vi "myRIO Main.vi"() -> ()   [LabVIEW 2014]
uses:
  Type Defs/VL6180X DEFS.ctl
  <vilib>/Analysis/baseanly.llb/Mean (DBL).vi
  <vilib>/MakerHub/LINX/Public/Utilities/Open Local.vi
  <vilib>/MakerHub/LINX/LMH-LINX.lvlib
  <vilib>/Analysis/NI_AALBase.lvlib
panel:
  in  "Speed Read":bool=TRUE
  out "Loop Rate (Hz)":u32
  in  "Offset":u8 format="%02x"
  out "Data out":u8 format="%02x"
  out "range":dbl
  out "Array":dbl[](array[numeric])
  out "min value":dbl
  out "max value":dbl
  in  "Samples to Avg":i32=10
  in  "milliseconds to wait":u32=20
  out "Sensor Error Code":u8
  in  "Stop":bool
  out "Distance":cluster{"Distance (mm)":u8, u8}(graph)
  # "0 = No error\n6 = early convergence estimate check failed\n7 = max convergence issue"
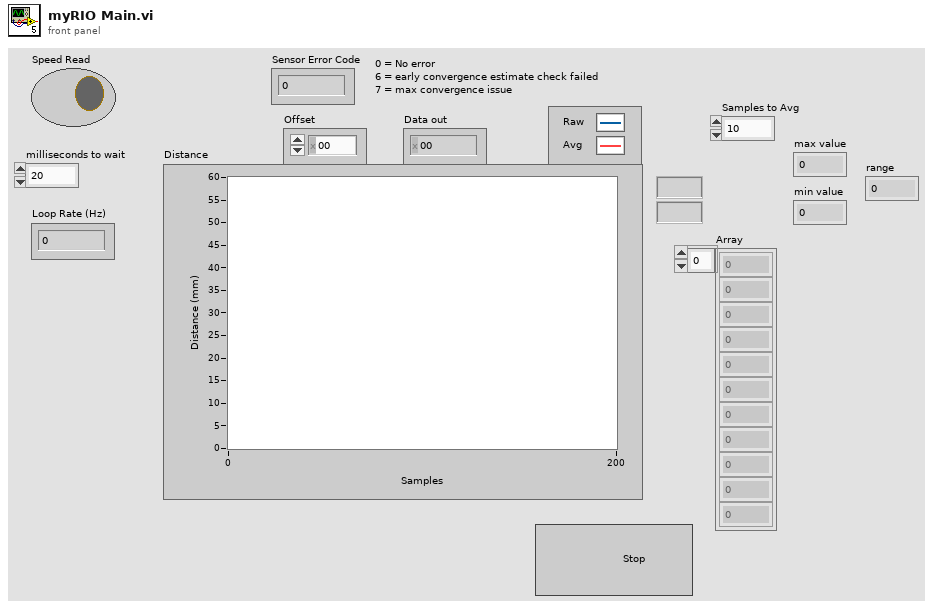
[diagram p1: front panel]
types:
  T1 = typedef "LMH-LINX.lvlib/LINX Ref.ctl" = cluster{"IO":T2, "Interface":T3, "LINX Device Config":T4}
  T2 = typedef "LMH-LINX.lvlib/Platform.ctl" = enum16{"Remote", "Local"}
  T3 = typedef "LMH-LINX.lvlib/Interface.ctl" = enum16{"Serial", "TCP"}
  T4 = typedef "LMH-LINX.lvlib/Device.lvlib/LINX Device Config.ctl" = cluster{"Interface":T3, "COM Port":refnum<visa-resource-name>, "TCP Configuration":T5, "Device Family":u8, "Device ID":u8, "Device Name":string, "TCP Ref":refnum<k5>, "Channels":T6}
  T5 = typedef "LMH-LINX.lvlib/Device.lvlib/TCP Config.ctl" = cluster{"IP Address":string, "Port":u16}
  T6 = typedef "LMH-LINX.lvlib/Channels.ctl" = cluster{"DI":u8[], "DO":u8[], "AI":u8[], "AO":u8[], "PWM":u8[], "QE":u8[], "UART":u8[], "I2C 2":u8[], "SPI":u8[], "CAN":u8[], "Servo":u8[], "AI Ref (V)":dbl, "AI Resolution (Bits)":u8, "AO Ref (V)":dbl, "AO Resolution (Bits)":u8}
  T7 = typedef "VL6180 Resource.ctl" = cluster{"LINX Resource":T1, "I2C Channel":u8, "I2C Slave Address":u8}
  T8 = typedef "VL6180X DEFS.ctl" = u16
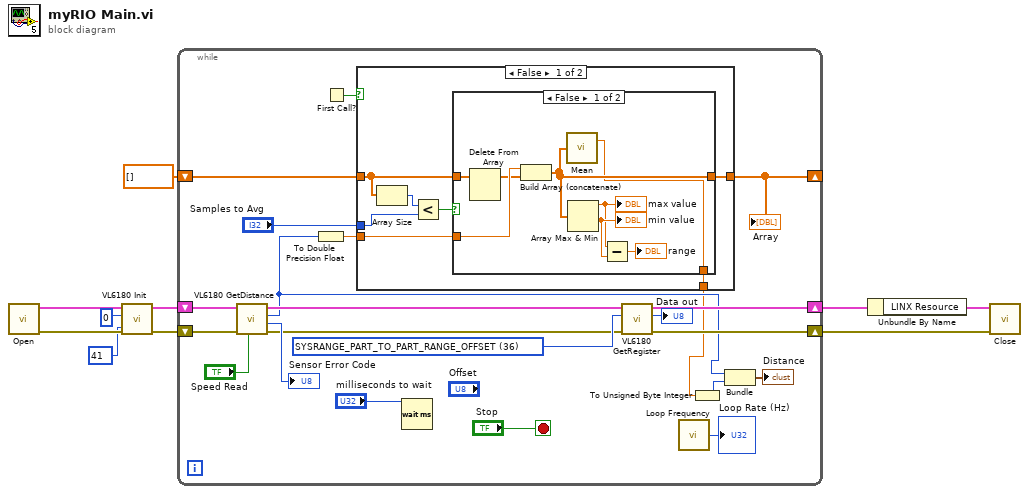
[diagram p0: block diagram]
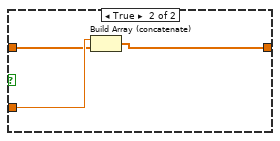
[diagram p2: hidden frame]
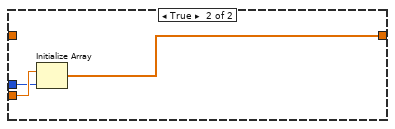
[diagram p3: hidden frame]
diagram:
  n1 = call-poly <vilib>:"Open.vi"() -> ("Error Out"=w9:errorcluster, "LINX Resource"=w10:T1)  [unwired: 9 in, 1 out]
  n2 = call "VL6180 Init.vi"("Error In"=w9, "I2C Slave Address (0)"=u8 41, "I2C Channel"=u8 0, "LINX Resource"=w10) -> ("Error Out"=w5:errorcluster, "VL6180 Resource"=w6:T7)  [unwired: 6 in]
  n3 = while {
    shift-right: [w22] -> w3
    shift-left: w6 -> [w32]
    shift-right: [w21] -> w4
    shift-left: w5 -> [w31]
    shift-right: [w24] -> _
    shift-left: dbl[] [] -> [w23]
    stop <- "Stop" stop-if-true
    w19 = T8 36 items=["IDENTIFICATION_MODEL_ID"=0, "IDENTIFICATION_MODEL_REV_MAJOR"=1, "IDENTIFICATION_MODEL_REV_MINOR"=2, "IDENTIFICATION_MODULE_REV_MAJOR"=3, "IDENTIFICATION_MODULE_REV_MINOR"=4, "IDENTIFICATION_DATE"=6, "IDENTIFICATION_TIME"=8, "SYSTEM_MODE_GPIO0"=16, "SYSTEM_MODE_GPIO1"=17, "SYSTEM_HISTORY_CTRL"=18, "SYSTEM_INTERRUPT_CONFIG_GPIO"=20, "SYSTEM_INTERRUPT_CLEAR"=21, "SYSTEM_FRESH_OUT_OF_RESET"=22, "SYSTEM_GROUPED_PARAMETER_HOLD"=23, "SYSRANGE_START"=24, "SYSRANGE_THRESH_HIGH"=25, "SYSRANGE_THRESH_LOW"=26, "SYSRANGE_INTERMEASUREMENT_PERIOD"=27, "SYSRANGE_MAX_CONVERGENCE_TIME"=28, "SYSRANGE_CROSSTALK_COMPENSATION_RATE"=30, "SYSRANGE_CROSSTALK_VALID_HEIGHT"=33, "SYSRANGE_EARLY_CONVERGENCE_ESTIMATE"=34, "SYSRANGE_PART_TO_PART_RANGE_OFFSET"=36, "SYSRANGE_RANGE_IGNORE_VALID_HEIGHT"=37, "SYSRANGE_RANGE_IGNORE_THRESHOLD"=38, "SYSRANGE_MAX_AMBIENT_LEVEL_MULT"=44, "SYSRANGE_RANGE_CHECK_ENABLES"=45, "SYSRANGE_VHV_RECALIBRATE"=46, "SYSRANGE_VHV_REPEAT_RATE"=49, "SYSALS_START"=56, "SYSALS_THRESH_HIGH"=58, "SYSALS_THRESH_LOW"=60, "SYSALS_INTERMEASUREMENT_PERIOD"=62, "SYSALS_ANALOGUE_GAIN"=63, "SYSALS_INTEGRATION_PERIOD"=64, "RESULT_RANGE_STATUS"=77, "RESULT_ALS_STATUS"=78, "RESULT_INTERRUPT_STATUS_GPIO"=79, "RESULT_ALS_VAL"=80, "RESULT_HISTORY_BUFFER"=82, "RESULT_RANGE_VAL"=98, "RESULT_RANGE_RAW"=100, "RESULT_RANGE_RETURN_RATE"=102, "RESULT_RANGE_REFERENCE_RATE"=104, "RESULT_RANGE_RETURN_SIGNAL_COUNT"=108, "RESULT_RANGE_REFERENCE_SIGNAL_COUNT"=112, "RESULT_RANGE_RETURN_AMB_COUNT"=116, "RESULT_RANGE_REFERENCE_AMB_COUNT"=120, "RESULT_RANGE_RETURN_CONV_TIME"=124, "RESULT_RANGE_REFERENCE_CONV_TIME"=128, "READOUT_AVERAGING_SAMPLE_PERIOD"=266, "FIRMWARE_BOOTUP"=281, "FIRMWARE_RESULT_SCALER"=288, "I2C_SLAVE_DEVICE_ADDRESS"=530, "INTERLEAVED_MODE_ENABLE"=675] ("VL6180X Constants")
    n4 = call "VL6180 GetDistance.vi"("Speed Read"="Speed Read", "error in (no error)"=w31, "VL6180 Resource in"=w32) -> ("error out"=w17:errorcluster, "Sensor Error Code"=→"Sensor Error Code":u8, "Distance (mm)"=w16:u8, "VL6180 Resource out"=w18:T7)  [unwired: 5 in]
    n5 = To Double Precision Float(number=w16) -> (double precision float=w26:dbl)
    n6 = First Call?() -> (First Call?: T/F=w27:bool)
    n7 = case shown="False" w27 {
      tunnel: w26 -> [w36 w53]
      tunnel: "Samples to Avg" -> [w37 w52]
      tunnel: [w34 w51] -> w24
      tunnel: w23 -> [w35 _]
      tunnel: [w33 _] -> w13
      frame False {
        n8 = Array Size(array=w35) -> (size(s)=w38:i32)
        n9 = Less?(x=w38, y=w37) -> (x < y?=w39:bool)
        n10 = case shown="False" w39 {
          tunnel: w36 -> [w46 w50]
          tunnel: w35 -> [w47 w49]
          tunnel: [w44 w48] -> w34
          tunnel: [w40 _] -> w33
          frame False {
            n11 = Delete From Array(array=w47) -> (array with subset deleted=w45:dbl[])  [unwired: 2 in, 1 out]
            n12 = Build Array (concatenate)(w46, w45) -> (w44:dbl[])
            n13 = call-poly <vilib>:"Mean.vi"("X"=w44) -> ("mean"=w40:dbl)  [unwired: 1 out]
            n14 = Array Max & Min(array=w44) -> (max value=w42:dbl, min value=w43:dbl)  [unwired: 2 out]
            "max value" <- w42
            "min value" <- w43
            n15 = Subtract(x=w42, y=w43) -> (x-y=→"range":dbl)
          }
          frame True {
            n16 = Build Array (concatenate)(w50, w49) -> (w48:dbl[])
          }
        }
      }
      frame True {
        n17 = Initialize Array(w53, w52) -> (w51:dbl[])
      }
    }
    "Array" <- w24
    n18 = Wait (ms)(milliseconds to wait="milliseconds to wait") -> ()  [unwired: 1 out]
    n19 = call "VL6180 GetRegister.vi"("error in"=w17, "VL6180X Constants"=w19, "VL6180 Resource"=w18) -> ("error out"=w21:errorcluster, "Data out"=→"Data out":u8, "VL6180 Resource"=w22:T7)  [unwired: 6 in]
    n20 = call <vilib>:"Loop Frequency.vi"() -> ("Loop Rate (Hz)"=→"Loop Rate (Hz)":u32)
    n21 = To Unsigned Byte Integer(number=w13) -> (unsigned 8bit integer=w12:u8)
    n22 = Bundle("Distance (mm)"=w16, w12) -> (→"Distance":cluster{"Distance (mm)":u8, u8})  [unwired: 1 in]
  }
  n23 = Unbundle By Name(w3) -> ("LINX Resource"=w2:T1)
  n24 = call <vilib>:"Close.vi"("Error In"=w4, "LINX Resource"=w2) -> ()  [unwired: 9 in, 1 out]
